vi "Wait on chirps generation-Conditional.vi"(11 "Next State":T1) -> (0 "error out":errorcluster, 3 "Timed out waiting on Chirps generation":bool)   [LabVIEW 2020]
uses:
  Typedefs/Top level VI states.ctl
  Typedefs/Imaging Protocols enum.ctl
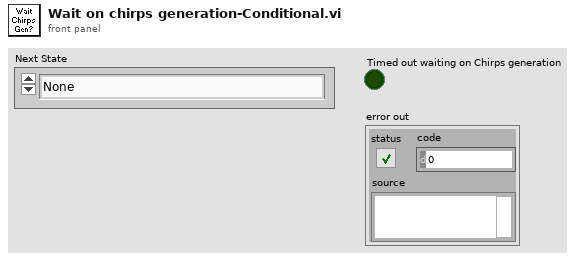
[diagram p1: front panel]
types:
  T1 = typedef "Top level VI states.ctl" = enum16{"None", "Initialise UI", "<STACK PROTOCOL STATES>", "AOL Zstack-START", "AOL Zstack-STOP", "Motor Zstack-START", "Motor Zstack-STOP", "<ACQUISITION PROTOCOL STATES> ", "Functional Acquisition-START", "Functional Acquisition-STOP", "Single Plane Acquisition-START", "Single Plane Acquisition-STOP", "Volume Acquisition-START", "Volume Acquisition-STOP", "<LIVE IMAGING PROTOCOL STATES>", "Live Imaging-START", "Live Imaging-STOP", "Live Plane Imaging-START", "Live Plane Imaging-STOP", "Live Volume Imaging-START", "Live Volume Imaging-STOP", "<MOVEMENT CORRECTION PROTOCOL STATES>", "EXIT"}
  T2 = typedef "Imaging Protocols enum.ctl" = enum16{"AOL Z-Stack", "Motor Z Stack", "Functional Acquisition", "Single Plane Acquisition", "Volume Acquisition", "Live Imaging", "Live Plane Imaging", "Live Volume Imaging"}
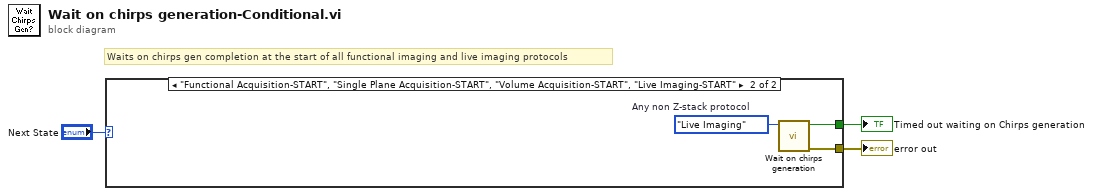
[diagram p0: block diagram]
diagram:
  # "Waits on chirps gen completion at the start of all functional imaging and live imaging protocols"
  n1 = case shown="\"Functional Acquisition-START\", \"Single Plane Acquisition-START\", \"Volume Acquisition-START\", \"Live Imaging-START\"" "Next State" {
    tunnel: [_ w6] -> w2
    tunnel: [_ w5] -> w3
    frame Default {
    }
    frame "Functional Acquisition-START", "Single Plane Acquisition-START", "Volume Acquisition-START", "Live Imaging-START" {
      w4 = Imaging_Protocols_enum."Live Imaging"  # Any non Z-stack protocol
      n2 = call "Wait on chirps generation.vi"("Imaging Protocol"=w4) -> ("error out"=w5:errorcluster, "Timed out waiting on Chirps generation"=w6:bool)  [unwired: 9 in]
    }
  }
  "error out" <- w3
  "Timed out waiting on Chirps generation" <- w2
